vi "Dependency Generate Parameters.vi"(8 "error in (no error)":errorcluster, 10 "Generated files in":path[][](array[path]), 11 "Project XML Editor in":refnum<class "Project XML Editor.lvclass">) -> (0 "error out":errorcluster, 2 "Dependency Parameters":T1[](array[typedef]), 3 "Project XML Editor out":refnum<class "Project XML Editor.lvclass">)   [LabVIEW 2019, in "Project XML Editor.lvclass"]
uses:
  Project XML Editor.lvclass
  TypeDefs/Dependency Parameters.ctl
  Project XML Editor.lvclass/Project XML Editor.ctl
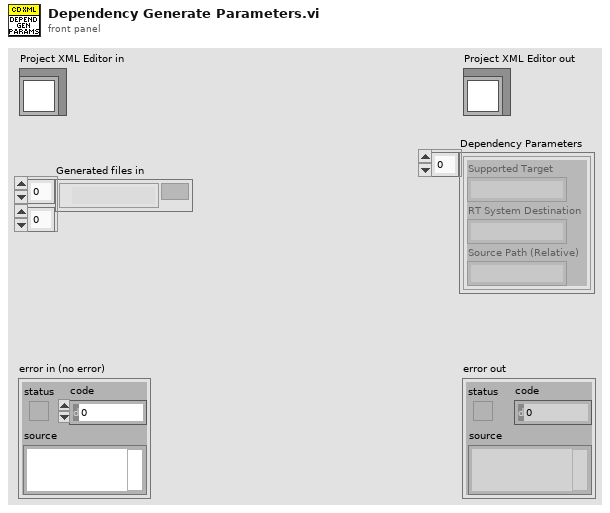
[diagram p1: front panel]
types:
  T1 = typedef "Project XML Editor.lvclass/Dependency Parameters.ctl" = cluster{"Supported Target":string, "RT System Destination":string, "Source Path (Relative)":string}
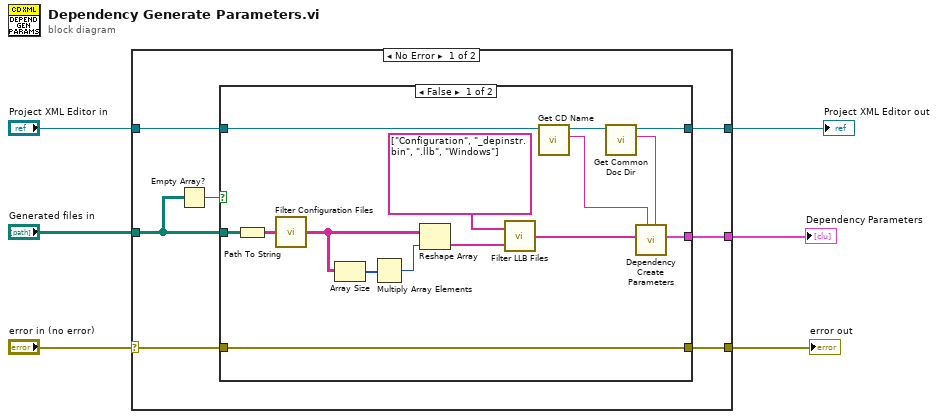
[diagram p0: block diagram]
diagram:
  n1 = case shown="No Error" "error in (no error)" {
    selector: "error in (no error)" -> [w7 w32]
    tunnel: [w8 w32] -> w5
    tunnel: [w12 w31] -> w3
    tunnel: "Project XML Editor in" -> [w13 w31]
    tunnel: "Generated files in" -> [w10 _]
    tunnel: [w11 _] -> w1
    frame No Error {
      n2 = Empty Array?(array=w10) -> (empty?=w9:bool)
      n3 = case shown="False" w9 {
        tunnel: w13 -> [w23 w30]
        tunnel: [w21 w30] -> w12
        tunnel: [w17 _] -> w11
        tunnel: w10 -> [w16 _]
        tunnel: [w15 w29] -> w8
        tunnel: w7 -> [w15 w29]
        frame False {
          n4 = Path To String(path=w16) -> (string=w26:string[][])
          n5 = call "Filter Configuration Files.vi"("Generated Files in"=w26) -> ("Generated Files out"=w25:string[][])
          n6 = Array Size(array=w25) -> (size(s)=w27:i32[])
          n7 = Multiply Array Elements(1:w27) -> (0:w28:i32)
          n8 = Reshape Array(w25, w28) -> (w24:string[])
          n9 = call "Filter LLB Files.vi"("Generated Files in"=w24, "Filter Array"=string[] ["Configuration", "_depinstr.bin", ".llb", "Windows"]) -> ("Generated Files out"=w20:string[])
          n10 = call "Get CD Name.vi"("Project XML Editor in"=w23) -> ("CD Name"=w19:string, "Project XML Editor out"=w22:refnum<class "Project XML Editor.lvclass">)  [unwired: 9 in]
          n11 = call "Get Common Doc Dir.vi"("Project XML Editor in"=w22) -> ("Common Doc Dir"=w18:string, "Project XML Editor out"=w21:refnum<class "Project XML Editor.lvclass">)  [unwired: 9 in]
          n12 = call "Dependency Create Parameters.vi"("Common Doc Dir"=w18, "CD Name"=w19, "Generated Files in"=w20) -> ("Dependency Parameters"=w17:T1[])  [unwired: 8 in]
        }
        frame True {
        }
      }
    }
    frame Error {
    }
  }
  "error out" <- w5
  "Project XML Editor out" <- w3
  "Dependency Parameters" <- w1
